vi "Check Drive Fault Error.vi"(1 "Map":map{string, dbl}(c390)) -> (0 "error out":errorcluster)   [LabVIEW 2024, in "UI.lvlib"]
uses:
  UI.lvlib
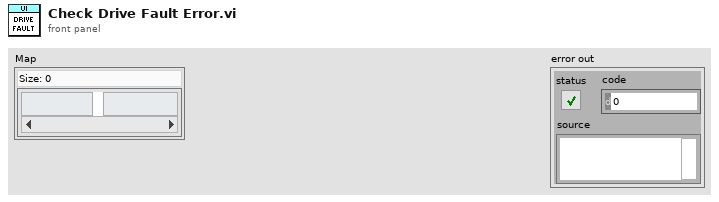
[diagram p1: front panel]
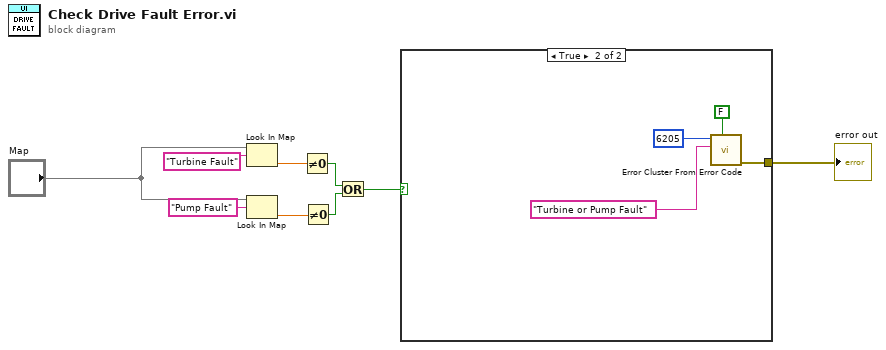
[diagram p0: block diagram]
diagram:
  n1 = Look In Map(map="Map", key="Turbine Fault") -> (value=w6:dbl)  [unwired: 1 in, 1 out]
  n2 = Look In Map(map="Map", key="Pump Fault") -> (value=w5:dbl)  [unwired: 1 in, 1 out]
  n3 = Not Equal To 0?(x=w6) -> (x != 0?=w4:bool)
  n4 = Not Equal To 0?(x=w5) -> (x != 0?=w3:bool)
  n5 = Or(x=w4, y=w3) -> (x .or. y?=w2:bool)
  n6 = case shown="True" w2 {
    tunnel: [_ w11] -> w9
    frame False {
    }
    frame True {
      n7 = call <vilib>:"Error Cluster From Error Code.vi"("show call chain? (False)"=FALSE, "error message (\"\")"="Turbine or Pump Fault" ("error message (\"\")"), "error code (0)"=6205) -> ("error out"=w11:errorcluster)  [unwired: 6 in]
    }
  }
  "error out" <- w9
